vi "initialise.vi"(8 "error in (no error)":errorcluster, 11 "DL090603DAQmxOnOffEmissionSensor in":refnum<class "DetectorDL090603DAQmxOnOff.lvclass">=refnum) -> (0 "error out":errorcluster, 3 "DL090603DAQmxOnOffEmissionSensor out":refnum<class "DetectorDL090603DAQmxOnOff.lvclass">)   [LabVIEW 2010, in "DetectorDL090603DAQmxOnOff.lvclass"]
doc: "The dynamic dispatch-version of this VI initalises the plug-in object by allocating and initalising any dynamic resources need."
uses:
  DetectorDL090603DAQmxOnOff.lvclass
  GenericDetector/GenericDetector/GenericDetector.lvclass
  DetectorDL090603DAQmxOnOff.lvclass/DetectorDL090603DAQmxOnOff.ctl
  DigitalOut/DigitalOutDL110325DAQmx/DigitalOutDL110325DAQmx/DigitalOutDL110325DAQmx.lvclass
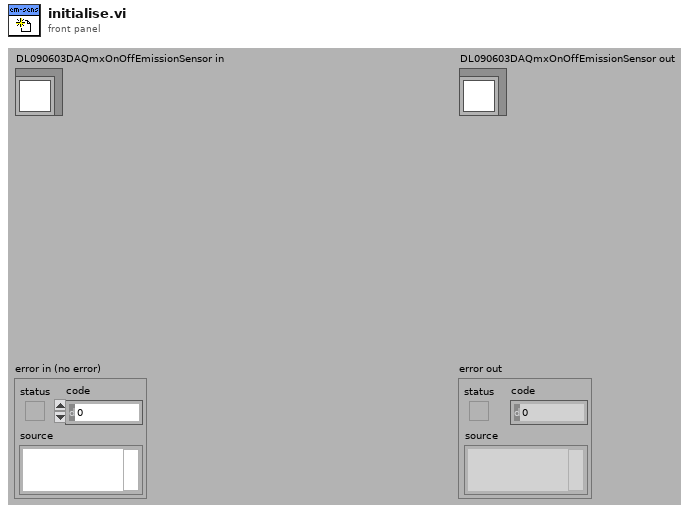
[diagram p1: front panel]
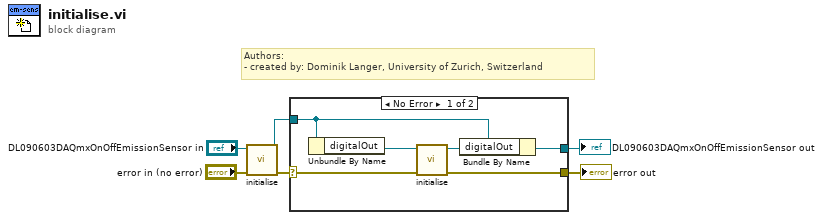
[diagram p0: block diagram]
diagram:
  # "Authors: \n- created by: Dominik Langer, University of Zurich, Switzerland"
  n1 = call-parent "initialise.vi"("error in (no error)"="error in (no error)", "GenericPlugin in"="DL090603DAQmxOnOffEmissionSensor in") -> ("error out"=w4:errorcluster, "GenericPlugin out"=w3:refnum<class "DetectorDL090603DAQmxOnOff.lvclass">)  [unwired: 8 out]
  n2 = case shown="No Error" w4 {
    selector: w4 -> [w12 w13]
    tunnel: w3 -> [w10 w14]
    tunnel: [w7 w13] -> w2
    tunnel: [w9 w14] -> w1
    frame No Error {
      n3 = Unbundle By Name(w10) -> ("digitalOut"=w11:refnum<class "DigitalOutDL110325DAQmx.lvclass">)
      n4 = call-dynamic "initialise.vi"("error in (no error)"=w12, "DAQmxDigitalOut in"=w11) -> ("error out"=w7:errorcluster, "DAQmxDigitalOut out"=w8:refnum<class "DigitalOutDL110325DAQmx.lvclass">)  [unwired: 8 out]
      n5 = Bundle By Name(cluster=w10, "digitalOut"=w8) -> (w9:refnum<class "DetectorDL090603DAQmxOnOff.lvclass">)
    }
    frame Error {
    }
  }
  "error out" <- w2
  "DL090603DAQmxOnOffEmissionSensor out" <- w1
